vi "replaces_instances.vi"(8 "error in (no error)":errorcluster, 9 "instances":refnum<data-value>[](array[refnum]), 10 "Base Class (LabVIEW Object)":refnum<class>, 11 "Lookup Service in":refnum<class "Lookup Service.lvclass">) -> (0 "error out":errorcluster, 3 "Lookup Service out":refnum<class "Lookup Service.lvclass">)   [LabVIEW 2014, in "LVCOOOP.lvlib" / "Lookup API.lvlib" / "Lookup Service.lvclass"]
uses:
  Lookup Service.lvclass
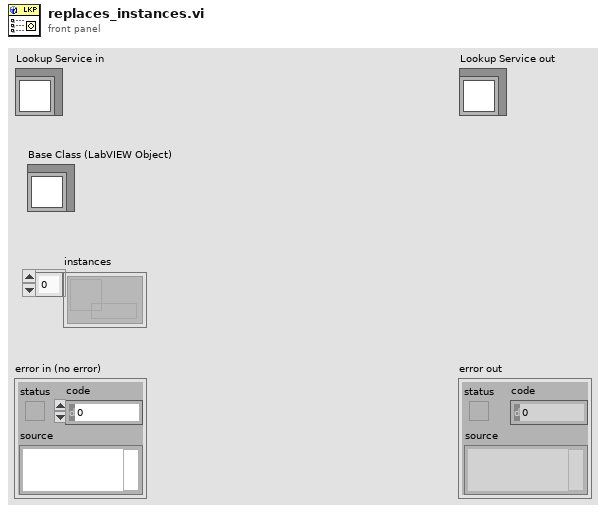
[diagram p1: front panel]
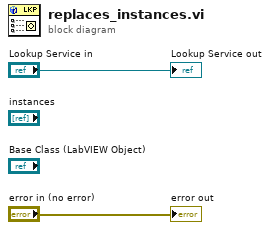
[diagram p0: block diagram]
diagram:
  "error out" <- "error in (no error)"
  "Lookup Service out" <- "Lookup Service in"
